vi "backup2.vi"() -> ()   [LabVIEW 2018]
panel:
  in  "stop":bool
  out "unsigned byte array 2":u8[](array[numeric]) format="%x"
  out "unsigned byte array":u8[](array[numeric])
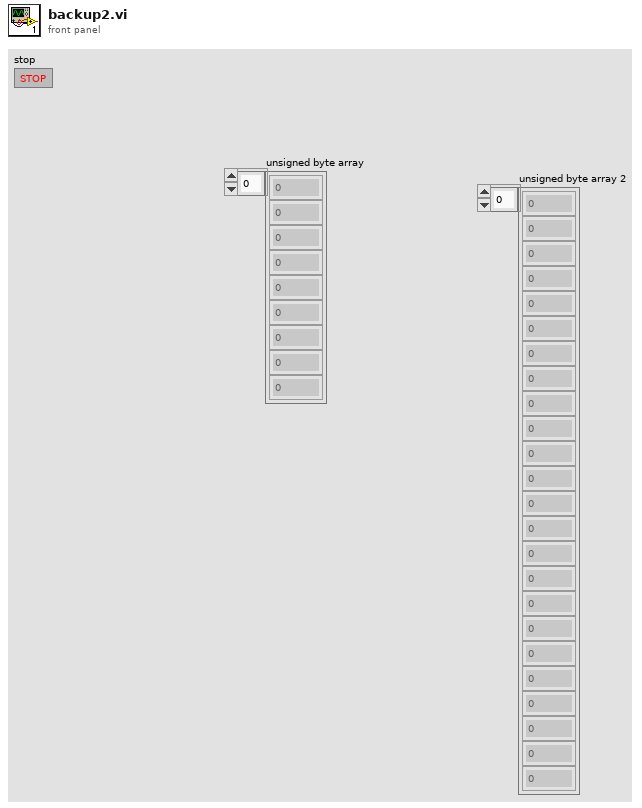
[diagram p1: front panel]
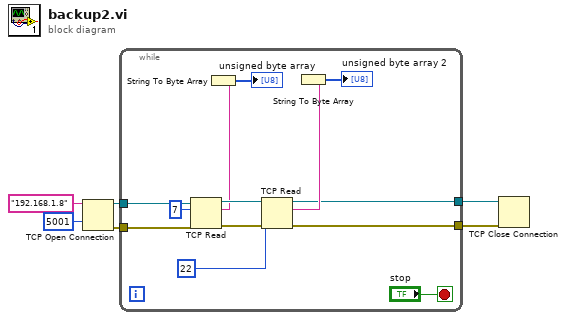
[diagram p0: block diagram]
diagram:
  n1 = TCP Open Connection(address="192.168.1.8", remote port or service name=u16 5001) -> (connection ID=w6:refnum<k5>, error out=w5:errorcluster)  [unwired: 3 in]
  n2 = while {
    tunnel: w6 -> [w19]
    tunnel: w5 -> [w17]
    tunnel: [w9] -> w2
    tunnel: [w8] -> w1
    stop <- "stop" stop-if-true
    n3 = TCP Read(connection ID=w19, bytes to read=7, error in (no error)=w17) -> (connection ID out=w18:refnum<k5>, data out=w13:string, error out=w16:errorcluster)  [unwired: 2 in]
    n4 = String To Byte Array(string=w13) -> (unsigned byte array=→"unsigned byte array":u8[])
    n5 = TCP Read(connection ID=w18, bytes to read=22, error in (no error)=w16) -> (connection ID out=w8:refnum<k5>, data out=w10:string, error out=w9:errorcluster)  [unwired: 2 in]
    n6 = String To Byte Array(string=w10) -> (unsigned byte array=→"unsigned byte array 2":u8[])
  }
  n7 = TCP Close Connection(connection ID=w1, error in (no error)=w2) -> ()  [unwired: 1 in, 2 out]
